vi "(定制产品)设置PWM频率和占空比.vi"(5 "占空比(0~1)":dbl, 7 "频率":dbl, 8 "错误输入":errorcluster caption="错误输入（无错误）", 10 "通道号":i32, 11 "设备句柄入":i32) -> (0 "错误输出":errorcluster, 3 "设备句柄":i32=1, 4 "实际占空比":dbl, 6 "实际频率":dbl)   [LabVIEW 2011]
uses:
  dll/em9636.dll
panel:
  in  "超时毫秒":i32=1000
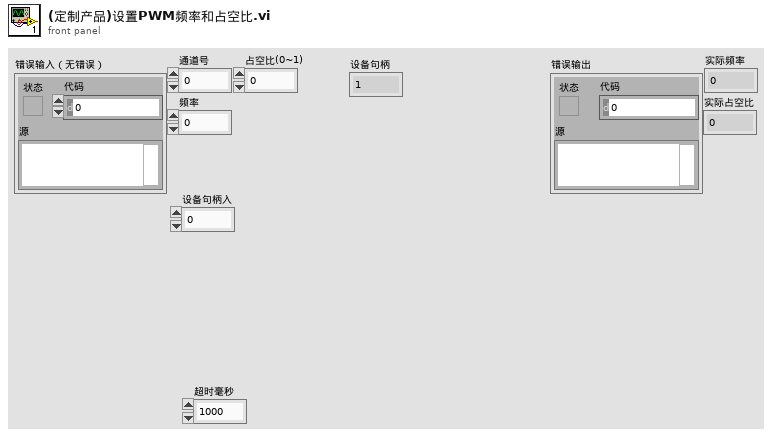
[diagram p1: front panel]
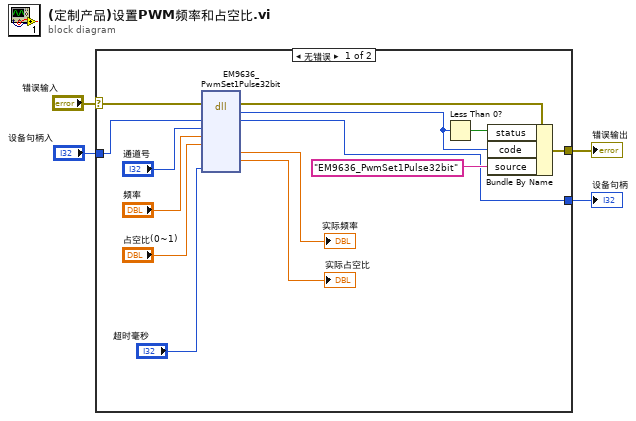
[diagram p0: block diagram]
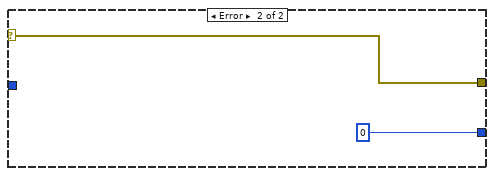
[diagram p2: hidden frame]
diagram:
  n1 = case shown="无错误" "错误输入" {
    selector: "错误输入" -> [w18 w20]
    tunnel: [w14 w20] -> w3
    tunnel: [w10 0 ("错误")] -> w2
    tunnel: "设备句柄入" -> [w12 _]
    frame No Error {
      n2 = dll-call lib="PTH1abs Eèµ éç LABVIEWæºVI(v2.0)EM9636BD)EM9636BDè°ç¨APIå½æ°æ¹æ³éè®¯ä¾ç¨EM9636_demo_labview2011dll\nem9636.dll" fn="EM9636_PwmSet1Pulse32bit"(error in=w18, "设备句柄"=w12, "通道号只能为1"="通道号", "频率，最小为0.01Hz"="频率", "占空比(0~1)"="占空比(0~1)", "超时毫秒"="超时毫秒") -> (error out=w16:errorcluster, "错误"=w13:i32, "设备句柄"=w10:i32, "实际频率"=→"实际频率":dbl, "实际占空比"=→"实际占空比":dbl)  [unwired: 8 in, 1 out]
      n3 = Less Than 0?(x=w13) -> (x < 0?=w15:bool)
      n4 = Bundle By Name(cluster=w16, "status"=w15, "code"=w13, "source"="EM9636_PwmSet1Pulse32bit") -> (w14:errorcluster)
    }
    frame Error {
    }
  }
  "错误输出" <- w3
  "设备句柄" <- w2
